vi "zoom_hit.vi"(7 "refVI":refnum<vi>, 8 "error in":errorcluster, 11 "data_in":T1 {"config"."updateTime" format="%#_g ms"; "config"."lowPass" format="%#_g Hz"; "config"."highPass" format="%#_g Hz"; "config"."cutoff" format="%#_g dB"; "config"."preTrigger" format="%#_g ms"; "config"."thr" format="%#_g N"; "config"."duration" format="%#_g s"; "config"."rate" min=1652.0 max=51200.0 format="%#_g Hz"}) -> (0 "error out":errorcluster, 3 "data_out":T1 {"config"."updateTime" format="%#_g ms"; "config"."lowPass" format="%#_g Hz"; "config"."highPass" format="%#_g Hz"; "config"."cutoff" format="%#_g dB"; "config"."preTrigger" format="%#_g ms"; "config"."thr" format="%#_g N"; "config"."duration" format="%#_g s"; "config"."rate" min=1652.0 max=51200.0 format="%#_g Hz"})   [LabVIEW 2018]
uses:
  results_data.ctl
  MainFGV/Settings/Advanced/AdvancedConfig.ctl
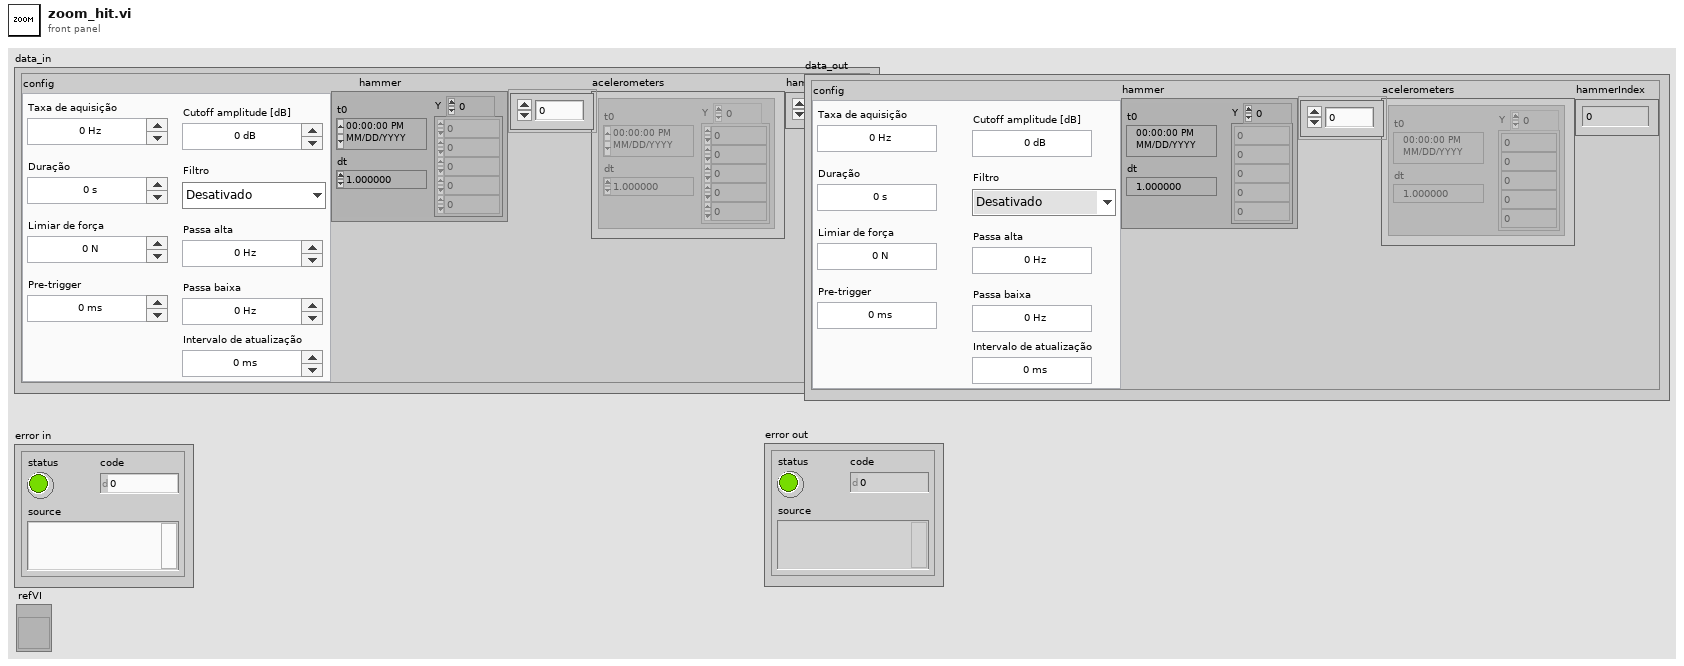
[diagram p1: front panel]
types:
  T1 = typedef "results_data.ctl" = cluster{"config":T2, "hammer":waveform(dbl), "acelerometers":waveform(dbl)[], "hammerIndex":i32}
  T2 = typedef "AdvancedConfig.ctl" = cluster{"rate":dbl, "duration":dbl, "thr":dbl, "preTrigger":dbl, "cutoff":dbl, "Filtro":enum16{"Desativado", "Passa banda", "Passa alta", "Passa baixa"}, "highPass":dbl, "lowPass":dbl, "updateTime":dbl}
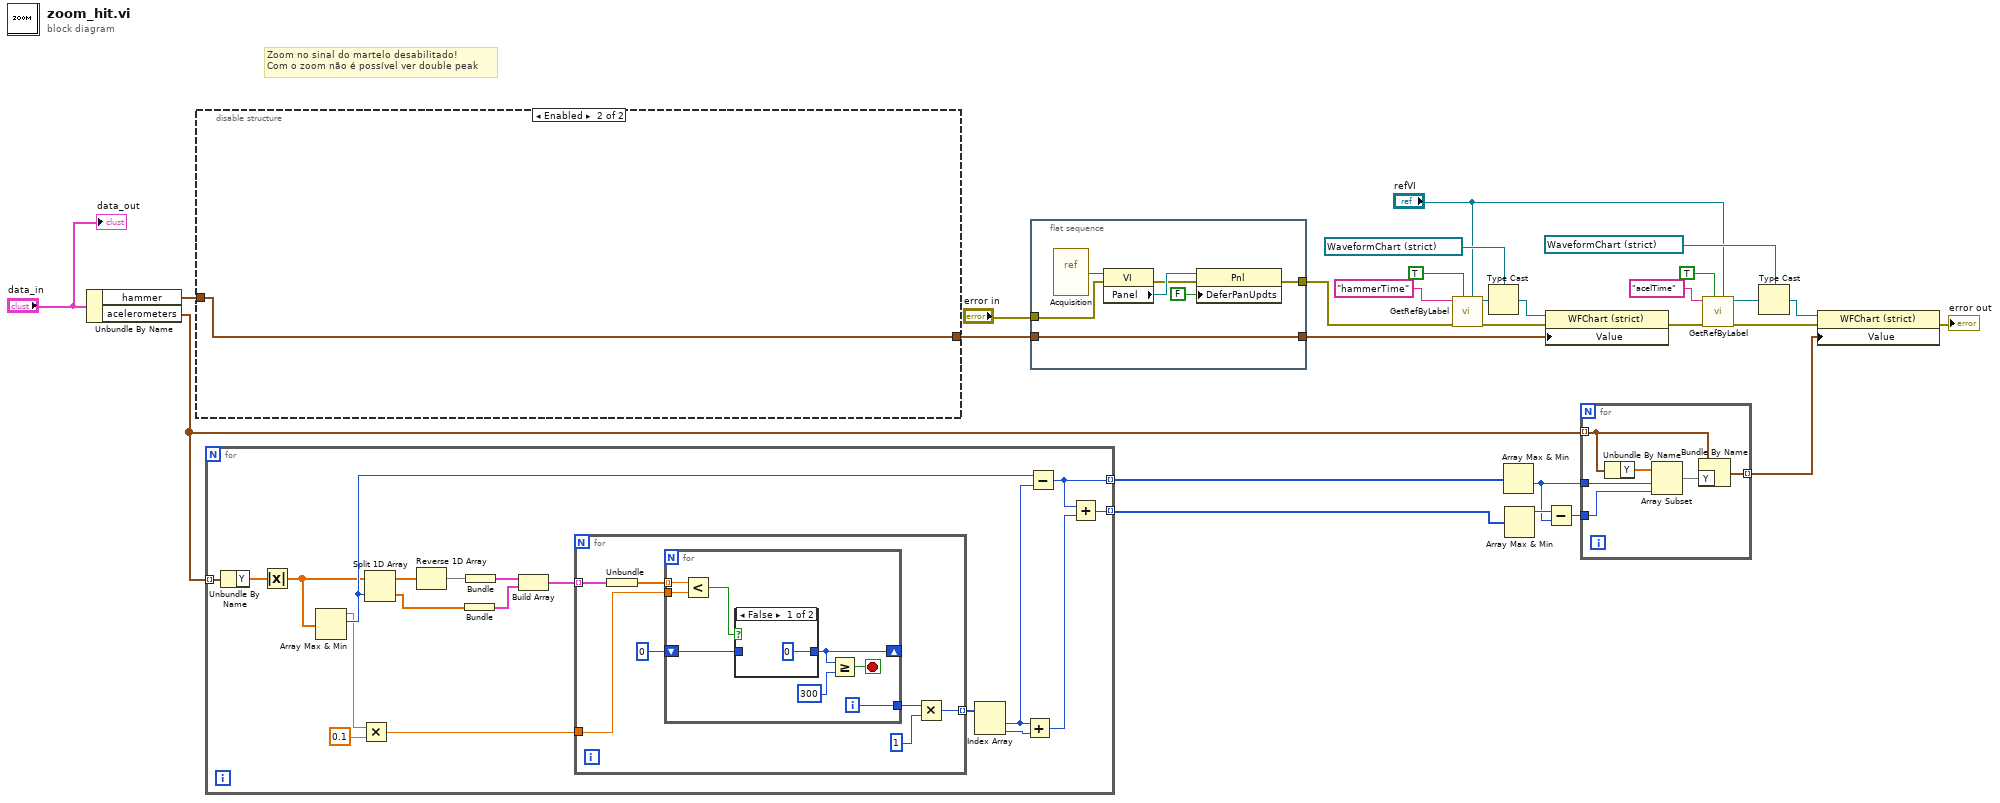
[diagram p0: block diagram]
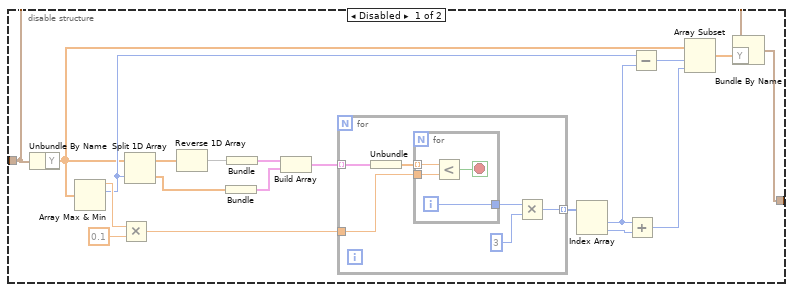
[diagram p2: hidden frame]
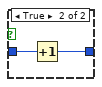
[diagram p3: hidden frame]
diagram:
  # "Zoom no sinal do martelo desabilitado!\nCom o zoom não é possível ver double peak"
  n1 = Unbundle By Name("data_in") -> ("hammer"=w27:waveform(dbl), "acelerometers"=w23:waveform(dbl)[])
  n2 = disable-structure shown="Enabled" {
    disable-tunnel: w27 -> [w30 w58]
    disable-tunnel: [w29 w58] -> w1
    frame Disabled {
      n3 = Unbundle By Name(w30) -> ("Y"=w32:dbl[])
      n4 = Array Max & Min(array=w32) -> (max value=w41:dbl, max index (indices)=w36:i32)  [unwired: 2 out]
      n5 = Multiply(x=w41, y=0.1) -> (x*y=w39:dbl)
      n6 = Split 1D Array(array=w32, index=w36) -> (first subarray=w47:dbl[], second subarray=w45:dbl[])
      n7 = Reverse 1D Array(array=w47) -> (reversed array=w46:dbl[])
      n8 = Bundle(w45) -> (w43:cluster{dbl[]})  [unwired: 1 in]
      n9 = Bundle(w46) -> (w44:cluster{dbl[]})  [unwired: 1 in]
      n10 = Build Array(w44, w43) -> (w42:cluster{dbl[]}[])
      n11 = for {
        tunnel: w42 -> [w53] mode=indexing
        tunnel: w39 -> [w51]
        tunnel: [w48] -> w38 mode=indexing
        n12 = Unbundle(w53) -> (w52:dbl[])
        n13 = for {
          tunnel: w52 -> [w57] mode=indexing
          tunnel: w51 -> [w56]
          tunnel: [w54] -> w50
          i -> [w54]
          stop <- w55 stop-if-true
          n14 = Less?(x=w57, y=w56) -> (x < y?=w55:bool)
        }
        n15 = Multiply(x=w50, y=3) -> (x*y=w48:i32)
      }
      n16 = Index Array(array=w38) -> (element #1=w35:i32, element #2=w37:i32)  [unwired: 2 in]
      n17 = Add(x=w35, y=w37) -> (x+y=w33:i32)
      n18 = Subtract(x=w36, y=w35) -> (x-y=w34:i32)
      n19 = Array Subset(array=w32, index=w34, length=w33) -> (w31:dbl[])
      n20 = Bundle By Name(cluster=w30, "Y"=w31) -> (w29:waveform(dbl))
    }
    frame Enabled {
    }
  }
  n21 = for {
    tunnel: w23 -> [w64] mode=indexing
    tunnel: [w60] -> w26 mode=indexing
    tunnel: [w59] -> w25 mode=indexing
    n22 = Unbundle By Name(w64) -> ("Y"=w63:dbl[])
    n23 = Absolute Value(x=w63) -> (abs(x)=w62:dbl[])
    n24 = Array Max & Min(array=w62) -> (max value=w71:dbl, max index (indices)=w76:i32)  [unwired: 2 out]
    n25 = Multiply(x=w71, y=0.1) -> (x*y=w73:dbl)
    n26 = Split 1D Array(array=w62, index=w76) -> (first subarray=w65:dbl[], second subarray=w67:dbl[])
    n27 = Reverse 1D Array(array=w65) -> (reversed array=w66:dbl[])
    n28 = Bundle(w67) -> (w69:cluster{dbl[]})  [unwired: 1 in]
    n29 = Bundle(w66) -> (w68:cluster{dbl[]})  [unwired: 1 in]
    n30 = Build Array(w68, w69) -> (w70:cluster{dbl[]}[])
    n31 = for {
      tunnel: w70 -> [w84] mode=indexing
      tunnel: w73 -> [w82]
      tunnel: [w79] -> w74 mode=indexing
      n32 = Unbundle(w84) -> (w83:dbl[])
      n33 = for {
        tunnel: w83 -> [w92] mode=indexing
        tunnel: w82 -> [w91]
        tunnel: [w90] -> w81
        shift-right: [w87] -> _
        shift-left: 0 ("y") -> [w88]
        i -> [w90]
        stop <- w85 stop-if-true
        n34 = Less?(x=w92, y=w91) -> (x < y?=w89:bool)
        n35 = case shown="False" w89 {
          tunnel: w88 -> [_ w95]
          tunnel: [0 ("y") w94] -> w87
          frame False {
          }
          frame True {
            n36 = Increment(x=w95) -> (x+1=w94:i32)
          }
        }
        n37 = Greater Or Equal?(x=w87, y=300) -> (x >= y?=w85:bool)
      }
      n38 = Multiply(x=w81, y=1) -> (x*y=w79:i32)
    }
    n39 = Index Array(array=w74) -> (element #1=w77:i32, element #2=w75:i32)  [unwired: 2 in]
    n40 = Add(x=w77, y=w75) -> (x+y=w61:i32)
    n41 = Subtract(x=w76, y=w77) -> (x-y=w60:i32)
    n42 = Add(x=w60, y=w61) -> (x+y=w59:i32)
  }
  n43 = flat-sequence {
    tunnel: "error in" -> [w98]
    tunnel: [w97] -> w3
    tunnel: [w96] -> w2
    tunnel: w1 -> [w96]
    frame #0 {
      n44 = vi-ref "Acquisition.vi"() -> (w102:refnum<vi>)
      n45 = property class="VI"(reference=w102, error in=w98) -> (error out=w100:errorcluster, "Panel"=w101:refnum<vi>)  [unwired: 1 out]
      n46 = property class="Pnl"(reference=w101, error in=w100, "DeferPanUpdts"=FALSE ("Defer Panel Updates")) -> (error out=w97:errorcluster)  [unwired: 1 out]
    }
  }
  n47 = call "GetRefByLabel.vi"("refVI"="refVI", "InsideTab"=TRUE, "error in"=w3, "Label"="hammerTime") -> ("error out"=w16:errorcluster, "Ctl Refnum"=w17:refnum<vi>)  [unwired: 5 in, 1 out]
  n48 = Type Cast(type=refnum<vi> refnum ("hammerTime"), x=w17) -> (*(type *) &x=w15:refnum<vi>)
  n49 = Array Max & Min(array=w26) -> (min value=w22:i32)  [unwired: 3 out]
  n50 = Array Max & Min(array=w25) -> (max value=w24:i32)  [unwired: 3 out]
  n51 = property class="WFChart (strict)"(reference=w15, error in=w16, "Value"=w2) -> (error out=w11:errorcluster)  [unwired: 1 out]
  n52 = Subtract(x=w24, y=w22) -> (x-y=w21:i32)
  n53 = for {
    tunnel: w23 -> [w107] mode=indexing
    tunnel: w22 -> [w105]
    tunnel: w21 -> [w104]
    tunnel: [w103] -> w7 mode=indexing
    n54 = Unbundle By Name(w107) -> ("Y"=w106:dbl[])
    n55 = Array Subset(array=w106, index=w105, length=w104) -> (w108:dbl[])
    n56 = Bundle By Name(cluster=w107, "Y"=w108) -> (w103:waveform(dbl))
  }
  n57 = call "GetRefByLabel.vi"("refVI"="refVI", "InsideTab"=TRUE, "error in"=w11, "Label"="acelTime") -> ("error out"=w8:errorcluster, "Ctl Refnum"=w14:refnum<vi>)  [unwired: 5 in, 1 out]
  n58 = Type Cast(type=refnum<vi> refnum ("acelTime"), x=w14) -> (*(type *) &x=w9:refnum<vi>)
  n59 = property class="WFChart (strict)"(reference=w9, error in=w8, "Value"=w7) -> (error out=→"error out":errorcluster)  [unwired: 1 out]
  "data_out" <- "data_in"
